vi "DLConnect.vi"(8 "error in (no error)":errorcluster, 10 "ON/OFF":bool=TRUE, 11 "Control in":refnum<class "Control.lvclass">) -> (0 "error out":errorcluster, 3 "Control out":refnum<class "Control.lvclass">)   [LabVIEW 2015]
uses:
  Control.lvclass
  dependecies/ControlsVIs/Clusters-def/Message type in control.ctl
  dependecies/ControlsVIs/Clusters-def/command cluster.ctl
  dependecies/ControlsVIs/Clusters-def/List-of-commands.ctl
  Message/Message.lvclass
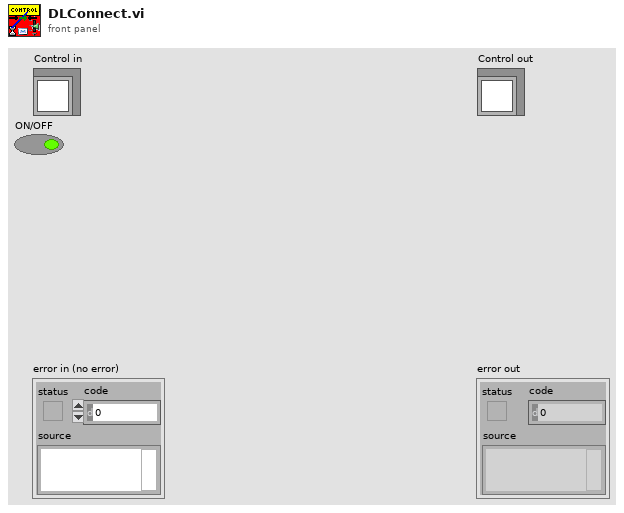
[diagram p1: front panel]
types:
  T1 = typedef "List-of-commands.ctl" = string
  T2 = typedef "command cluster.ctl" = cluster{"command name":string, "data":variant}
  T3 = typedef "Message type in control.ctl" = string
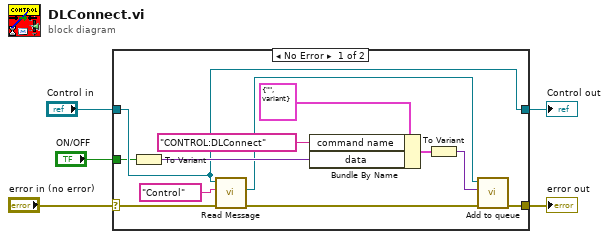
[diagram p0: block diagram]
diagram:
  n1 = case shown="No Error" "error in (no error)" {
    selector: "error in (no error)" -> [w8 w19]
    tunnel: [w7 w19] -> w4
    tunnel: [w9 w18] -> w2
    tunnel: "Control in" -> [w9 w18]
    tunnel: "ON/OFF" -> [w6 _]
    frame No Error {
      n2 = To Variant(anything=w6) -> (Variant=w16:variant)
      n3 = call-dynamic "Read Message.vi"("error in (no error)"=w8, "Message type"=T3 "Control", "Control in"=w9) -> ("error out"=w11:errorcluster, "Message.lvclass"=w12:refnum<class "Message.lvclass">)  [unwired: 6 in, 1 out]
      n4 = Bundle By Name(cluster=T2 {"command name"="", "data"=variant} ("input cluster"), "command name"=T1 "CONTROL:DLConnect" ("Commands"), "data"=w16) -> (w14:T2)
      n5 = To Variant(anything=w14) -> (Variant=w15:variant)
      n6 = call "Add to queue.vi"("error in (no error)"=w11, "Data"=w15, "Message in"=w12) -> ("error out"=w7:errorcluster)  [unwired: 7 in, 1 out]
    }
    frame Error {
    }
  }
  "error out" <- w4
  "Control out" <- w2
